vi "ArgoDriveScalingDemo.vi"() -> ()   [LabVIEW 2019]
uses:
  ArgosLib/ArgosLib.lvlib
panel:
  in  "Scale":dbl=0.2 format="%#_13g"
  out "Sat 2":cluster{"Array":dbl[], dbl[]}[](graph)
  out "Sat":cluster{"Array":dbl[], dbl[]}[](graph)
  in  "Array":dbl[](array[numeric])
  out "RawDiff":dbl
  out "SatDiff":dbl
  out "Right_Motor":dbl
  out "Left_Motor":dbl
  out "Right_Motor_Say":dbl
  out "Left_Motor_Sat":dbl
  in  "Turning":dbl(slide) scale=-1.0..1.0
  in  "Power":dbl(slide) scale=-1.0..1.0
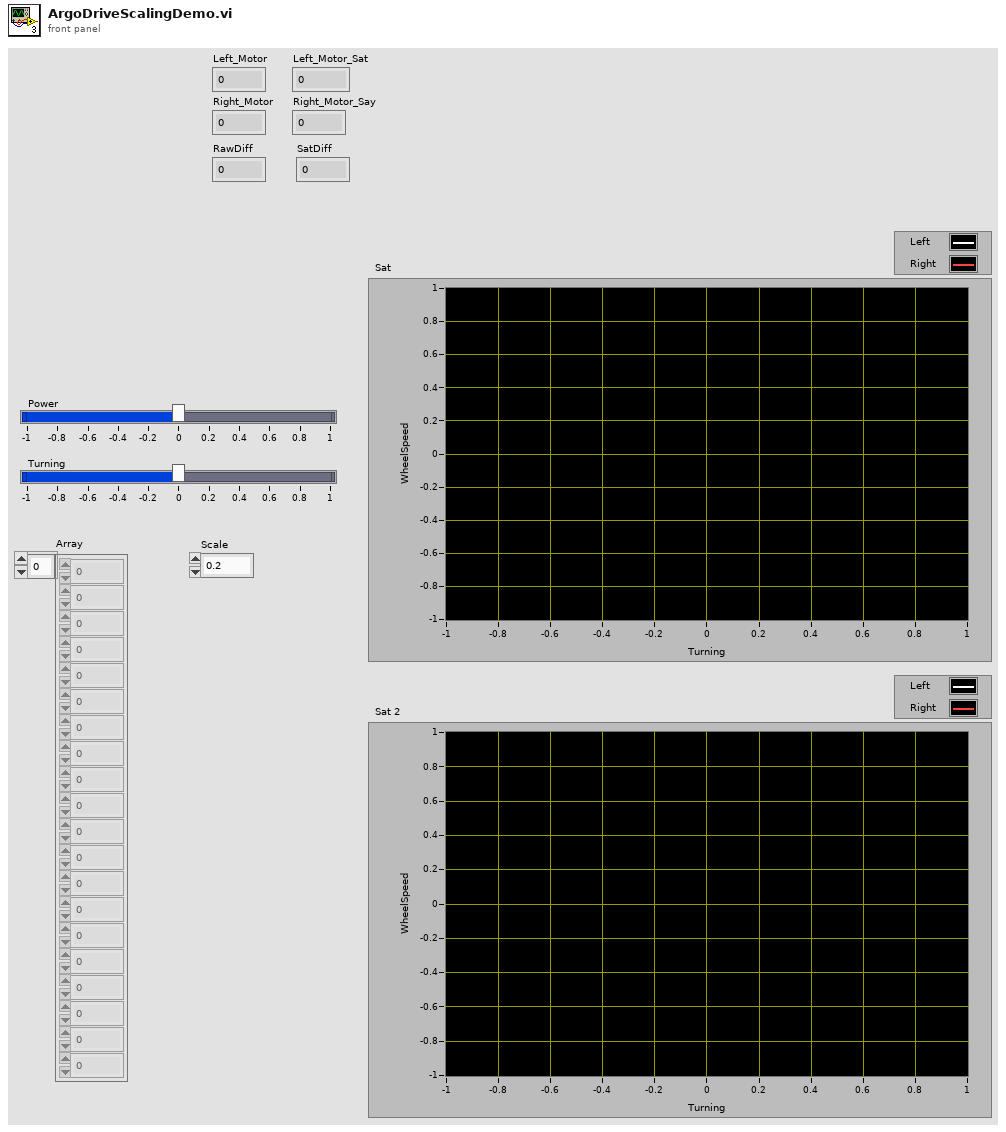
[diagram p1: front panel]
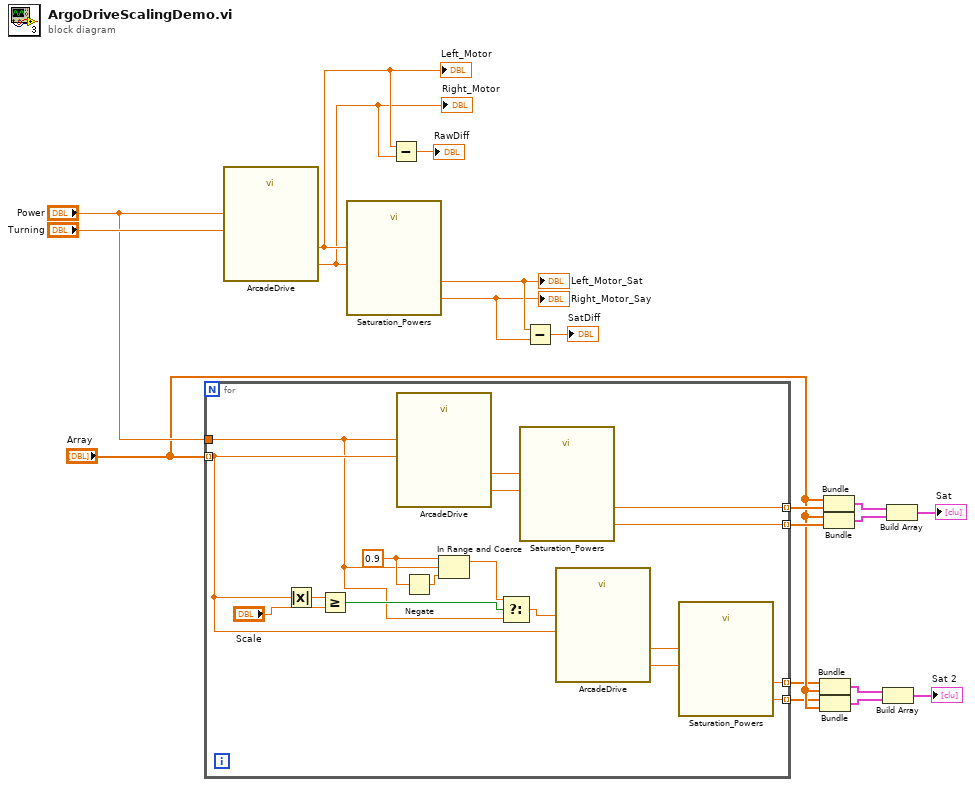
[diagram p0: block diagram]
diagram:
  n1 = for {
    tunnel: "Array" -> [w28] mode=indexing
    tunnel: "Power" -> [w21]
    tunnel: [w34] -> w11 mode=indexing
    tunnel: [w33] -> w10 mode=indexing
    tunnel: [w30] -> w2 mode=indexing
    tunnel: [w29] -> w1 mode=indexing
    w26 = 0.9 ("upper limit")
    n2 = Absolute Value(x=w28) -> (abs(x)=w20:dbl)
    n3 = Greater Or Equal?(x=w20, y="Scale") -> (x >= y?=w23:bool)
    n4 = call "ArcadeDrive.vi"("Turning"=w28, "Power"=w21) -> ("Right_Motor"=w36:dbl, "Left_Motor"=w35:dbl)  [unwired: 8 in]
    n5 = Negate(x=w26) -> (-x=w25:dbl)
    n6 = In Range and Coerce(upper limit=w26, x=w21, lower limit=w25) -> (coerced(x)=w22:dbl)  [unwired: 1 out]
    n7 = Select(t=w22, s=w23, f=w21) -> (s? t:f=w24:dbl)
    n8 = call "Saturation_Powers.vi"("Right_Motor"=w36, "Left_Motor"=w35) -> ("Right_Motor_Sat"=w33:dbl, "Left_Motor_Sat"=w34:dbl)  [unwired: 8 in]
    n9 = call "ArcadeDrive.vi"("Turning"=w28, "Power"=w24) -> ("Right_Motor"=w31:dbl, "Left_Motor"=w32:dbl)  [unwired: 8 in]
    n10 = call "Saturation_Powers.vi"("Right_Motor"=w31, "Left_Motor"=w32) -> ("Right_Motor_Sat"=w29:dbl, "Left_Motor_Sat"=w30:dbl)  [unwired: 8 in]
  }
  n11 = call "ArcadeDrive.vi"("Turning"="Turning", "Power"="Power") -> ("Right_Motor"=w14:dbl, "Left_Motor"=w15:dbl)  [unwired: 8 in]
  "Left_Motor" <- w15
  "Right_Motor" <- w14
  n12 = call "Saturation_Powers.vi"("Right_Motor"=w14, "Left_Motor"=w15) -> ("Right_Motor_Sat"=w17:dbl, "Left_Motor_Sat"=w18:dbl)  [unwired: 8 in]
  "Left_Motor_Sat" <- w18
  "Right_Motor_Say" <- w17
  n13 = Subtract(x=w15, y=w14) -> (x-y=→"RawDiff":dbl)
  n14 = Subtract(x=w18, y=w17) -> (x-y=→"SatDiff":dbl)
  n15 = Bundle(w2, "Array"="Array") -> (w4:cluster{dbl[], "Array":dbl[]})  [unwired: 1 in]
  n16 = Bundle(w1, "Array"="Array") -> (w5:cluster{dbl[], "Array":dbl[]})  [unwired: 1 in]
  n17 = Bundle("Array"="Array", w11) -> (w9:cluster{"Array":dbl[], dbl[]})  [unwired: 1 in]
  n18 = Bundle("Array"="Array", w10) -> (w8:cluster{"Array":dbl[], dbl[]})  [unwired: 1 in]
  n19 = Build Array(w4, w5) -> (→"Sat 2":cluster{dbl[], "Array":dbl[]}[])
  n20 = Build Array(w9, w8) -> (→"Sat":cluster{"Array":dbl[], dbl[]}[])
